vi "LoadProjectRecursively.vi"(8 "error in (no error)":errorcluster, 10 "Project ref in":refnum<vi>, 11 "Application in":refnum<vi>) -> (0 "error out":errorcluster, 1 "VI Refs":refnum<vi>[](array[refnum]), 2 "Project ref out":refnum<vi>, 3 "Application out":refnum<vi>)   [LabVIEW 2017]
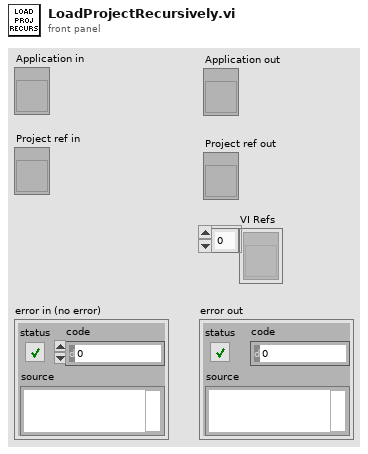
[diagram p1: front panel]
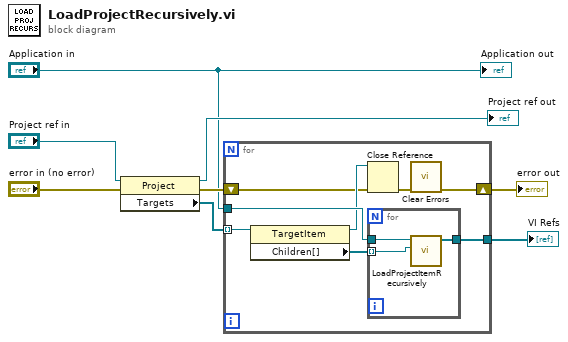
[diagram p0: block diagram]
diagram:
  n1 = property class="Project"(reference="Project ref in", error in="error in (no error)") -> (reference out=→"Project ref out":refnum<vi>, error out=w4:errorcluster, "Targets"=w6:refnum<vi>[])
  n2 = for {
    tunnel: w6 -> [w16] mode=indexing
    tunnel: "Application in" -> [w15]
    tunnel: [w14] -> w8
    shift-right: [w9] -> w3
    shift-left: w4 -> [w11]
    n3 = property class="TargetItem"(reference=w16) -> (reference out=w12:refnum<vi>, "Children[]"=w13:refnum<vi>[])  [unwired: 1 in, 1 out]
    n4 = Close Reference(reference=w12, error in (no error)=w11) -> (error out=w10:errorcluster)
    n5 = for {
      tunnel: w15 -> [w19]
      tunnel: [w18] -> w14
      tunnel: w13 -> [w17] mode=indexing
      n6 = call "LoadProjectItemRecursively.vi"("ProjectItem In"=w17, "Application in"=w19) -> ("VIRefs"=w18:refnum<vi>[])  [unwired: 8 in, 1 out]
    }
    n7 = call <vilib>:"Clear Errors.vi"("error in (no error)"=w10) -> ("error out"=w9:errorcluster)  [unwired: 5 in, 1 out]
  }
  "VI Refs" <- w8
  "error out" <- w3
  "Application out" <- "Application in"
